vi "RT_stage_control.vi"() -> ()   [LabVIEW 2019]
uses:
  StageControl.ctl
  <vilib>/Platform/TimedLoop/XDataNode/timing_clust.ctl
  <vilib>/Platform/TimedLoop/XDataNode/nitl_modes.ctl
  <vilib>/Platform/TimedLoop/XDataNode/wakeup.ctl
  <vilib>/FPGAPlugInAG/myRIO-1900/niLvFpga_Open_myRIO-1900.vi
  <vilib>/rvi/interface/common/dynamic/niFpgaDynamicAddResources.vi
  <vilib>/Utility/error.llb/Error Cluster From Error Code.vi
  <vilib>/rvi/errors/niLvFpgaAdjustHostInterfaceError.vi
  <vilib>/FPGAPlugInAG/Dynamic/niLvFpga_Close_Dynamic.vi
  <vilib>/rvi/interface/nirviOpenFPGA/nirviOpenFPGA.xnode
  FPGA Bitfiles/studentchallenge_FPGATarget_FPGARADCWDAC3_gNVwU-DQYMc.lvbitx
  FPGA_R_ADC_W_DAC.vi
  <vilib>/rvi/interface/nirviReadWriteControl/nirviReadWriteControl.xnode
  <vilib>/Platform/TimedLoop/XDataNode/XDataNode.xnode
  <vilib>/rvi/interface/nirviCloseFPGA/nirviCloseFPGA.xnode
  <vilib>/Platform/TimedLoop/XDataNode/XDNodeRunTimeDep.lvlib
  NiFpgaLv.dll
  <vilib>/rvi/interface/Simulation/niFpgaSimulationCallBeginRW.vi
panel:
  out "X Position":dbl format="%.4g"
  out "X Control Signal [V]":dbl
  out "num refs":i16
  out "Home Direction Flag":bool
  in  "Y Relative Position [mm]":dbl format="%#_13g"
  in  "X Relative Position [mm]":dbl format="%#_13g"
  out "Encoder B Offset":i32
  out "Encoder A Offset":i32
  out "Ref":refnum<k20>
  in  "Start":bool
  out "Y Position":dbl format="%.4g"
  in  "Operation":T1
  in  "stop":bool
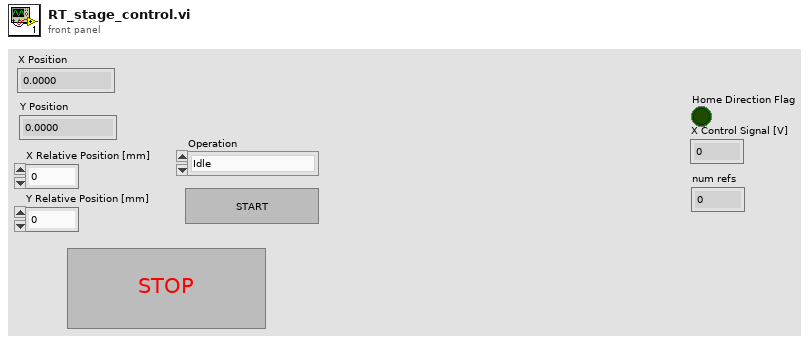
[diagram p1: front panel]
types:
  T1 = typedef "StageControl.ctl" = enum16{"Idle", "Home X", "Home Y"}
  T2 = typedef "XDNodeRunTimeDep.lvlib/timing_clust.ctl" = cluster{"Expected End [f-1]":u64, "Actual End [f-1]":u64, "Finished Late? [f-1]":bool, "Expected End [i-1]":u64, "Actual End [i-1]":u64, "Finished Late? [i-1]":bool, "Expected Start [i]":u64, "Actual Start [i]":u64, "Expected Start [f]":u64, "Actual Start [f]":u64, "Source Name":string, "Structure Name":string, "Period":i64, "Deadline":i64, "Offset":i64, "Start":i64, "Priority":i32, "Timeout":i32, "Mode":T3, "Wakeup Reason":T4, "Error":errorcluster, "Source Type":string, "Secondary Source Type":string, "Global End Time":u64, "Global Start Time":u64, "Frame Duration":u64, "Iteration Duration":u64, "Assigned CPU":i32, "I/O Scan Engine Mode":u32}
  T3 = typedef "XDNodeRunTimeDep.lvlib/nitl_modes.ctl" = enum32{"No Change", "Process missed periods, maintain original phase", "Discard missed periods, maintain original phase", "Process missed periods, ignore original phase", "Discard missed periods, ignore original phase"}
  T4 = typedef "XDNodeRunTimeDep.lvlib/wakeup.ctl" = enum32{"Normal", "Aborted", "Asynchronous wakeup", "Timing source error", "Timed loop error", "Timeout"}
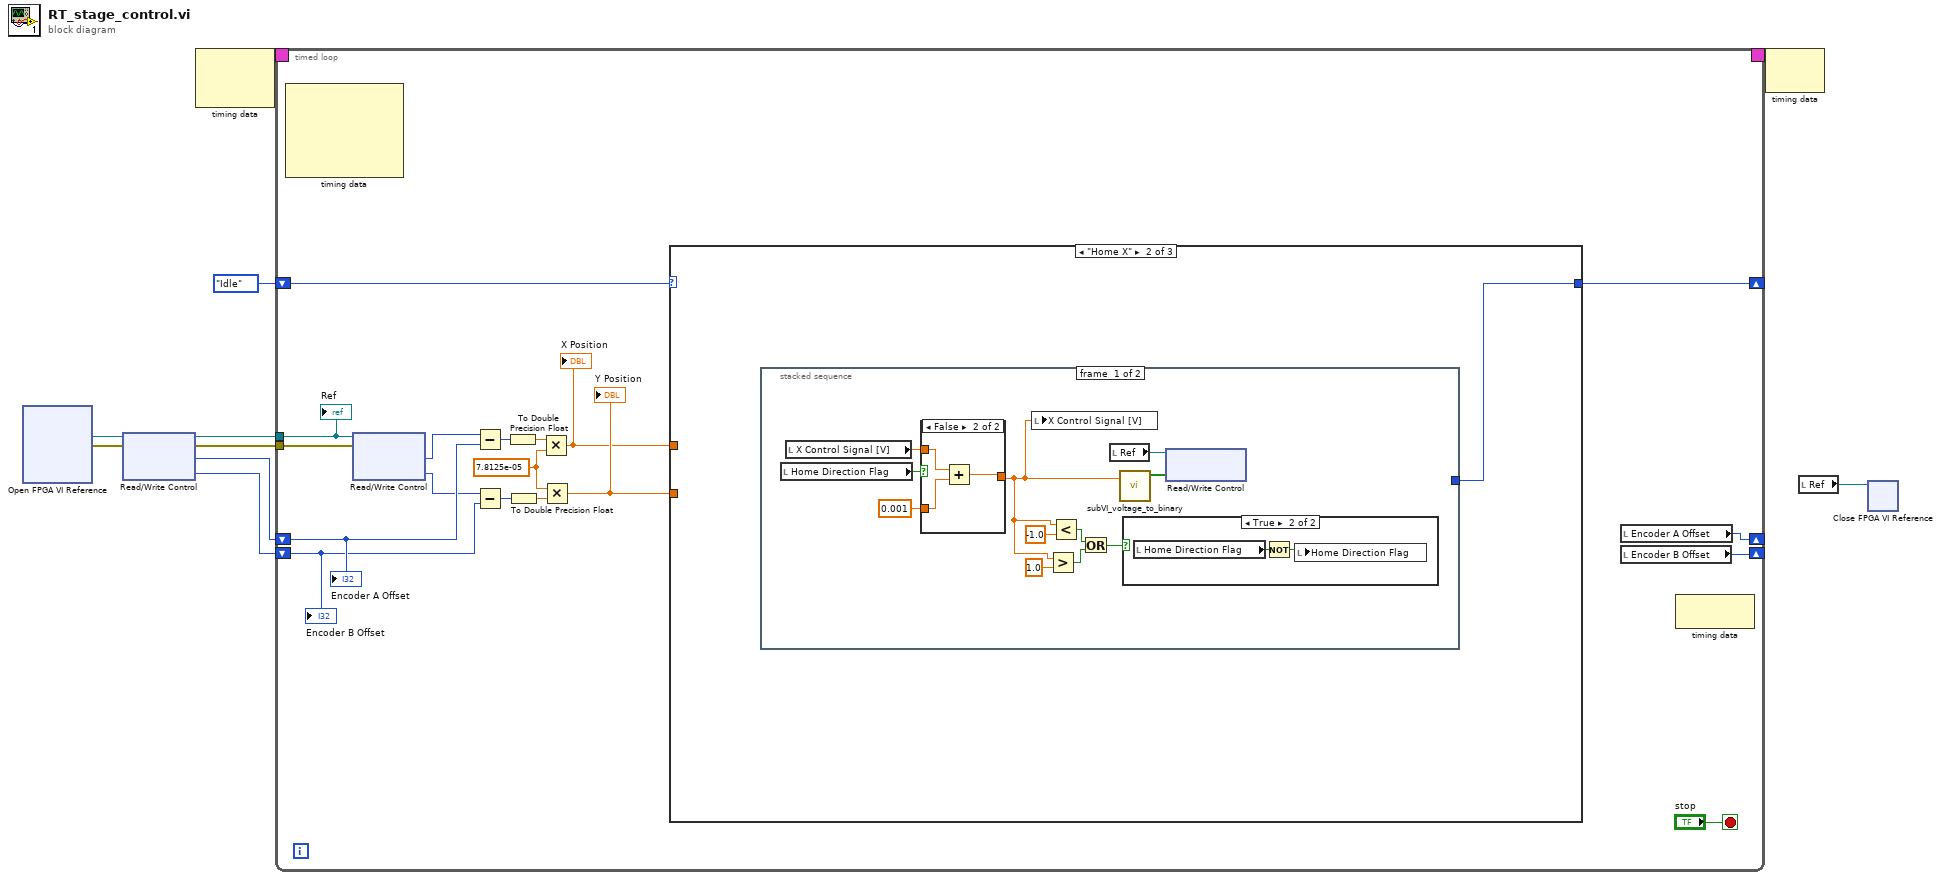
[diagram p0: block diagram]
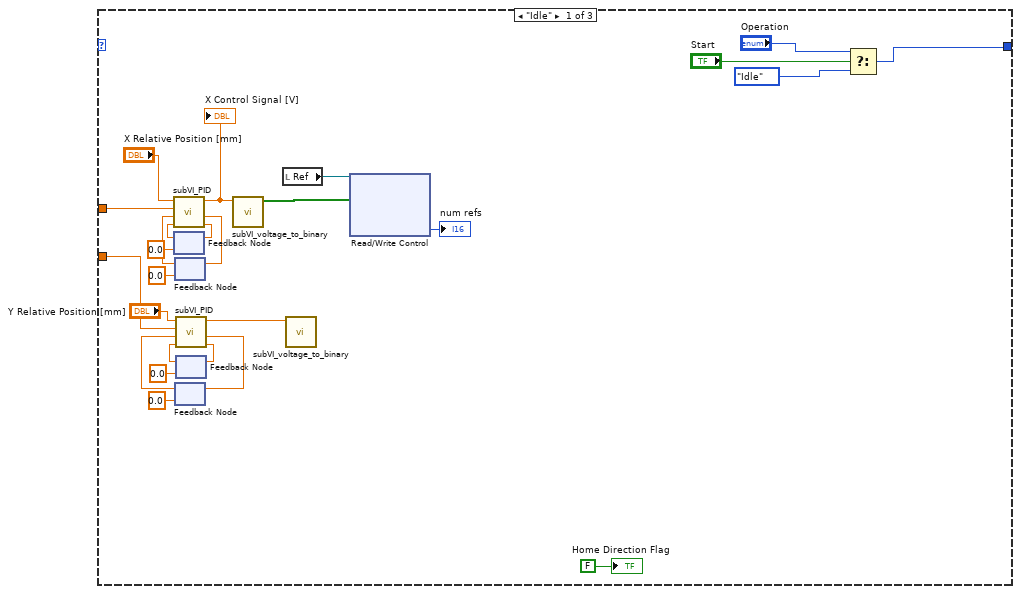
[diagram p2: hidden frame]
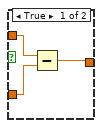
[diagram p4: hidden frame]
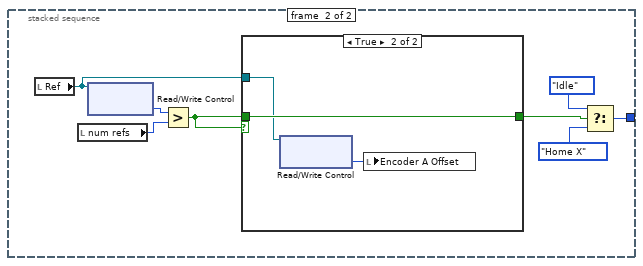
[diagram p5: hidden frame]
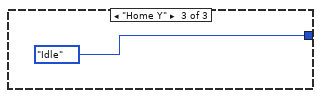
[diagram p7: hidden frame]
diagram:
  n1 = xnode "Open FPGA VI Reference"() -> ("FPGA VI Reference Out"=w8:refnum<k20>, "error out"=w7:errorcluster)  [unwired: 2 in]
  n2 = xnode "Read/Write Control"("FPGA VI Reference In"=w8, "error in"=w7) -> ("FPGA VI Reference Out"=w6:refnum<k20>, "error out"=w5:errorcluster, "Encoder A"=w4:i32, "Encoder B"=w3:i32)
  n3 = node-c288() -> (w10:T2)  [unwired: 2 in]
  n4 = timed-loop {
    shift-right: [w14] -> _
    shift-left: w4 -> [w19]
    timing: w10 -> [_]
    timing-out: [_] -> w9
    shift-right: [w13] -> _
    shift-left: w3 -> [w17]
    tunnel: w6 -> [w27]
    tunnel: w5 -> [w26]
    shift-right: [w16] -> _
    shift-left: StageControl."Idle" ("Enum 2") -> [w12]
    stop <- "stop" stop-if-true
    w21 = 7.8125e-05 ("y")
    n5 = node-c288() -> ()  [unwired: 1 in, 5 out]
    n6 = xnode "Read/Write Control"("FPGA VI Reference In"=w27, "error in"=w26) -> ("Encoder A"=w20:i32, "Encoder B"=w18:i32)  [unwired: 2 out]
    n7 = Subtract(x=w20, y=w19) -> (x-y=w24:i32)
    n8 = Subtract(x=w18, y=w17) -> (x-y=w23:i32)
    n9 = To Double Precision Float(number=w24) -> (double precision float=w25:dbl)
    n10 = To Double Precision Float(number=w23) -> (double precision float=w22:dbl)
    n11 = Multiply(x=w25, y=w21) -> (x*y=w11:dbl)
    "X Position" <- w11
    n12 = Multiply(x=w21, y=w22) -> (x*y=w15:dbl)
    "Y Position" <- w15
    n13 = case shown="\"Home X\"" w12 {
      tunnel: [w54 w55 StageControl."Idle" ("Enum 2")] -> w16
      tunnel: w11 -> [w49 _ _]
      tunnel: w15 -> [w48 _ _]
      frame "Idle" {
        n14 = feedback #1(0.0 ("Cumulative Error Out")) -> (w42:dbl)
        n15 = feedback #2(0.0 ("Error")) -> (w40:dbl)
        n16 = call "subVI_PID.vi"("Cumulative Error In"=w42, "Previous Error"=w40, "Encoder Position [mm]"=w49, "Desired Position [mm]"="X Relative Position [mm]") -> ("Cumulative Error Out"=w43:dbl, "Error"=w41:dbl, "Control Signal [V]"=w37:dbl)  [unwired: 5 in]
        "X Control Signal [V]" <- w37
        n17 = feedback-in #1(w43) -> ()
        n18 = feedback-in #2(w41) -> ()
        n19 = feedback #3(0.0 ("Error")) -> (w46:dbl)
        n20 = feedback #4(0.0 ("Cumulative Error Out")) -> (w44:dbl)
        n21 = call "subVI_PID.vi"("Cumulative Error In"=w44, "Previous Error"=w46, "Encoder Position [mm]"=w48, "Desired Position [mm]"="Y Relative Position [mm]") -> ("Cumulative Error Out"=w45:dbl, "Error"=w47:dbl, "Control Signal [V]"=w36:dbl)  [unwired: 5 in]
        n22 = feedback-in #3(w47) -> ()
        n23 = feedback-in #4(w45) -> ()
        n24 = call "subVI_voltage_to_binary.vi"("voltage"=w37) -> ("binary"=w35:bool[])  [unwired: 10 in]
        n25 = local read "Ref"() -> (w38:refnum<k20>)
        n26 = call "subVI_voltage_to_binary.vi"("voltage"=w36) -> ()  [unwired: 10 in, 1 out]
        n27 = xnode "Read/Write Control"("FPGA VI Reference In"=w38, "DAC 1 write"=w35) -> ("num refs"=→"num refs":i16)  [unwired: 2 in, 2 out]
        n28 = Select(t="Operation", s="Start", f=StageControl."Idle" ("Enum 2")) -> (s? t:f=w54:T1)
        "Home Direction Flag" <- FALSE
      }
      frame "Home X" {
        n29 = stacked-sequence {
          tunnel: [_ w78] -> w55
          frame #0 {
            n30 = local read "Home Direction Flag"() -> (w66:bool)
            n31 = local read "X Control Signal [V]"() -> (w65:dbl)
            n32 = case shown="False" w66 {
              tunnel: w65 -> [w71 w74]
              tunnel: 0.001 ("X Home Increment [V]") -> [w70 w73]
              tunnel: [w69 w72] -> w57
              frame True {
                n33 = Subtract(x=w71, y=w70) -> (x-y=w69:dbl)
              }
              frame False {
                n34 = Add(x=w74, y=w73) -> (x+y=w72:dbl)
              }
            }
            n35 = local write "X Control Signal [V]"(w57) -> ()
            n36 = Greater?(x=w57, y=1.0) -> (0:w59:bool)
            n37 = Less?(x=w57, y=-1.0) -> (x < y?=w60:bool)
            n38 = Or(x=w60, y=w59) -> (x .or. y?=w58:bool)
            n39 = local read "Ref"() -> (w63:refnum<k20>)
            n40 = call "subVI_voltage_to_binary.vi"("voltage"=w57) -> ("binary"=w64:bool[])  [unwired: 10 in]
            n41 = case shown="True" w58 {
              frame False {
              }
              frame True {
                n42 = local read "Home Direction Flag"() -> (w68:bool)
                n43 = Not(x=w68) -> (.not. x?=w67:bool)
                n44 = local write "Home Direction Flag"(w67) -> ()
              }
            }
            n45 = xnode "Read/Write Control"("FPGA VI Reference In"=w63, "DAC 1 write"=w64) -> ()  [unwired: 1 in, 2 out]
          }
          frame #1 {
            n46 = local read "Ref"() -> (w75:refnum<k20>)
            n47 = local read "num refs"() -> (w81:i16)
            n48 = xnode "Read/Write Control"("FPGA VI Reference In"=w75) -> ("num refs"=w82:i16)  [unwired: 1 in, 2 out]
            n49 = Greater?(x=w82, y=w81) -> (0:w76:bool)
            n50 = case shown="True" w76 {
              tunnel: [w83 w86] -> w77
              tunnel: w76 -> [w83 w86]
              tunnel: w75 -> [_ w85]
              frame False {
              }
              frame True {
                n51 = xnode "Read/Write Control"("FPGA VI Reference In"=w85) -> ("Encoder A"=w84:i32)  [unwired: 1 in, 2 out]
                n52 = local write "Encoder A Offset"(w84) -> ()
              }
            }
            n53 = Select(t=StageControl."Idle" ("Enum 2"), s=w77, f=StageControl."Home X" ("Enum 2")) -> (s? t:f=w78:T1)
          }
        }
      }
      frame "Home Y" {
      }
    }
    n54 = local read "Encoder A Offset"() -> (w14:i32)
    n55 = local read "Encoder B Offset"() -> (w13:i32)
    n56 = node-c288() -> ()  [unwired: 1 in, 1 out]
    "Ref" <- w27
    "Encoder A Offset" <- w19
    "Encoder B Offset" <- w17
  }
  n57 = node-c288(w9) -> ()  [unwired: 1 out]
  n58 = local read "Ref"() -> (w2:refnum<k20>)
  n59 = xnode "Close FPGA VI Reference"("FPGA VI Reference In"=w2) -> ()  [unwired: 1 in, 1 out]
